vi "Adapt and Merge Waveform.vi"(8 "Error":errorcluster, 9 "Raw Waveform":T1, 11 "WavBuf":refnum<class "WavBuf.lvclass">) -> (0 "Error Out":errorcluster, 3 "WavBuf Out":refnum<class "WavBuf.lvclass">, 5 "Left over Count":i32)   [LabVIEW 2025, in "WavBuf.lvclass"]
uses:
  WavBuf.lvclass
  Universal Controls/Waveform_Data.ctl
  WavBuf.lvclass/WavBuf.ctl
  Support/Waveform_Merge Waveforms.vi
  Support/Waveform_Resample with new dt.vi
  Support/Wavform_Select dt and check valid time.vi
  Support/t0_Valid.vi
  Support/tf_from t0.vi
  Support/t0_from tf.vi
  Support/Waveform_Read Write End Point Index.vi
  Support/Dbl Array_Linearize NAN values.vi
  Support/Timestamp_Convert Difference to dt Increments.vi
  <vilib>/Waveform/WDTOps.llb/Check for Equality.vi
  <vilib>/Waveform/WDTOps.llb/Waveform Duration.vi
  <vilib>/Waveform/WDTOps.llb/WDT Waveform Duration DBL.vi
  Support/Dbl Array_Place Line between points.vi
  Support/PointerArray_Offset.vi
panel:
  in  "Digital":bool
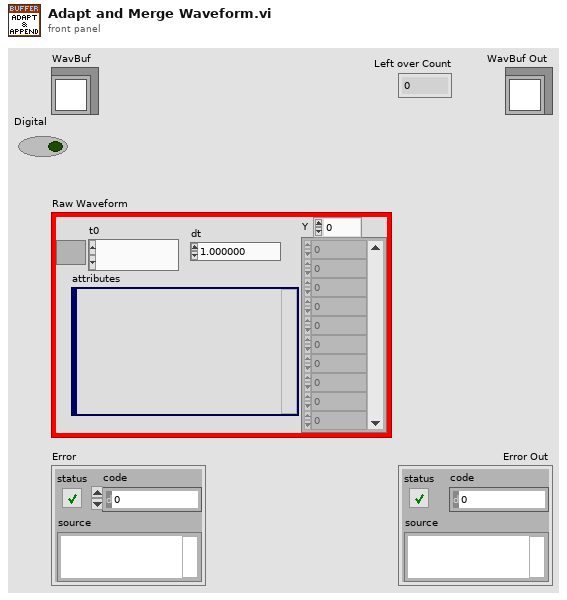
[diagram p1: front panel]
types:
  T1 = typedef "Waveform_Data.ctl" = waveform(dbl)
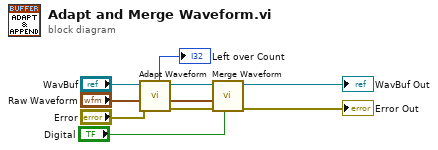
[diagram p0: block diagram]
diagram:
  n1 = call-dynamic "Adapt Waveform.vi"("Error"="Error", "Waveform"="Raw Waveform", "WavBuf"="WavBuf") -> ("Error Out"=w5:errorcluster, "Waveform Out"=w6:T1, "WavBuf Out"=w7:refnum<class "WavBuf.lvclass">, "Left over Count"=→"Left over Count":i32)  [unwired: 5 in]
  n2 = call "Merge Waveform.vi"("Digital"="Digital", "Error"=w5, "Waveform To Append"=w6, "WavBuf"=w7) -> ("Error Out"=→"Error Out":errorcluster, "WavBuf Out"=→"WavBuf Out":refnum<class "WavBuf.lvclass">)  [unwired: 6 in]
